vi "MICSD Get Calibration Data.vi"(8 "error in (no error)":errorcluster, 10 "Calibration Register":enum16{"INFO_D", "INFO_C"}(ring), 11 "VISA Resource Name":refnum<visa-resource-name>) -> (0 "error out":errorcluster, 1 "Calibration Data":u8[](array[numeric]) format="%02x", 3 "dup VISA Resource Name":refnum<visa-resource-name>)   [LabVIEW 2020]
uses:
  <vilib>/Instr/_visa.llb/VISA Configure Serial Port (Instr).vi
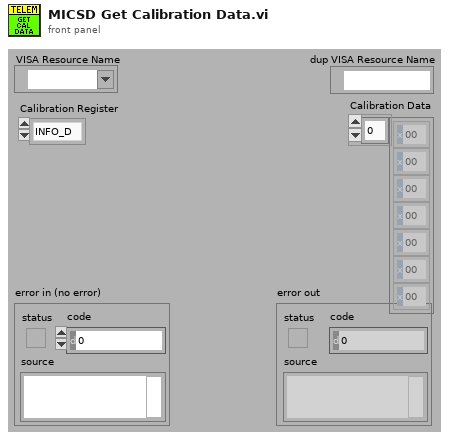
[diagram p1: front panel]
types:
  T1 = cluster{"Command Token":u8, "Length":u16, "Pack Data":u8[]}
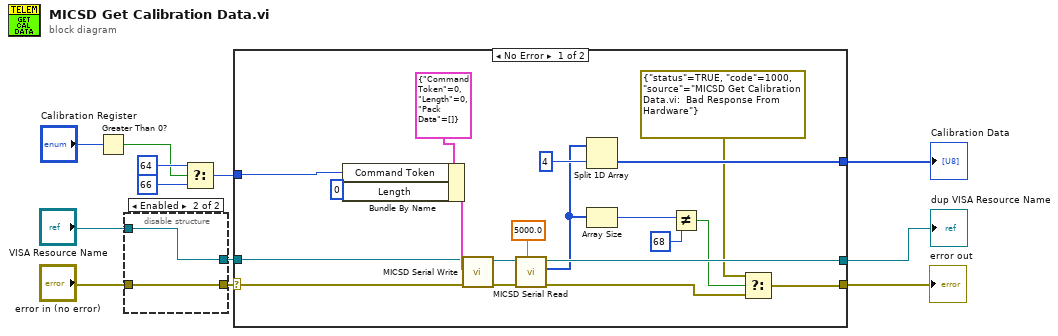
[diagram p0: block diagram]
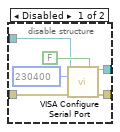
[diagram p2: hidden frame]
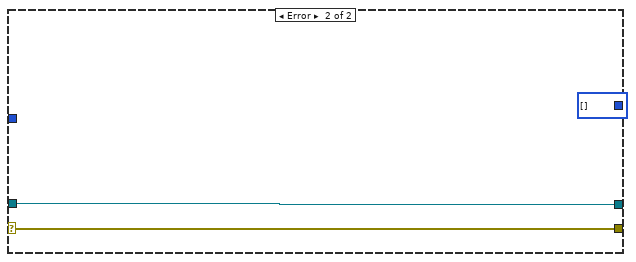
[diagram p3: hidden frame]
diagram:
  n1 = Greater Than 0?(x="Calibration Register") -> (x > 0?=w1:bool)
  n2 = disable-structure shown="Enabled" {
    disable-tunnel: [w16 w19] -> w12
    disable-tunnel: [w15 w20] -> w11
    disable-tunnel: "VISA Resource Name" -> [w14 w20]
    disable-tunnel: "error in (no error)" -> [w13 w19]
    frame Disabled {
      n3 = call-poly "VISA Configure Serial Port"("VISA resource name"=w14, "Enable Termination\nChar (T)"=FALSE ("Enable Termination\nChar (T)"), "baud rate (9600)"=u32 230400, "error in (no error)"=w13) -> ("VISA resource name out"=w15:refnum<visa-resource-name>, "error out"=w16:errorcluster)  [unwired: 10 in]
    }
    frame Enabled {
    }
  }
  n4 = Select(t=u8 64 ("Command Token"), s=w1, f=u8 66 ("Command Token")) -> (s? t:f=w5:u8)
  n5 = case shown="No Error" w12 {
    selector: w12 -> [w30 w42]
    tunnel: [w22 w42] -> w7
    tunnel: w11 -> [w31 w41]
    tunnel: [w35 w41] -> w8
    tunnel: [w28 u8[] []] -> w6
    tunnel: w5 -> [w29 _]
    frame No Error {
      n6 = Bundle By Name(cluster=T1 {"Command Token"=0, "Length"=0, "Pack Data"=[]} ("Write Data"), "Command Token"=w29, "Length"=u16 0) -> (w39:T1)
      n7 = call "MICSD Serial Write.vi"("error in (no error)"=w30, "Write Data"=w39, "VISA Resource Name"=w31) -> ("error out"=w34:errorcluster, "DUP Visa Resource Name"=w37:refnum<visa-resource-name>)  [unwired: 7 in]
      n8 = call "MICSD Serial Read.vi"("Timeout(mS)"=5000.0, "error in (no error)"=w34, "VISA Resource Name"=w37) -> ("error out"=w23:errorcluster, "Read Data"=w27:u8[], "DUP Visa Resource Name"=w35:refnum<visa-resource-name>)  [unwired: 6 in]
      n9 = Split 1D Array(array=w27, index=4) -> (second subarray=w28:u8[])  [unwired: 1 out]
      n10 = Array Size(array=w27) -> (size(s)=w21:i32)
      n11 = Not Equal?(x=w21, y=68) -> (x != y?=w25:bool)
      n12 = Select(t=errorcluster {"status"=TRUE, "code"=1000, "source"="MICSD Get Calibration Data.vi:  Bad Response From Hardware"} ("error IO"), s=w25, f=w23) -> (s? t:f=w22:errorcluster)
    }
    frame Error {
      (unwired) u16 0
    }
  }
  "dup VISA Resource Name" <- w8
  "error out" <- w7
  "Calibration Data" <- w6
